vi "Generate Non-Linear X-component.vi"(7 "Current Calibration Type":T1, 9 "Reso Phase correction factor":dbl, 10 "Start Delay (Ticks)":dbl, 11 "X Pixel Dimension":i32) -> (3 "Non-Linear X pixel Distribution (Linear for Galvo)":dbl[](array[numeric]))   [LabVIEW 2012]
uses:
  Custom Controls and Typedefs/CalibrationType.ctl
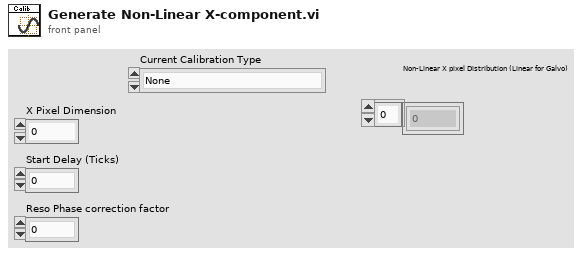
[diagram p1: front panel]
types:
  T1 = typedef "CalibrationType.ctl" = enum16{"None", "ImagingGalvoCalibration", "ImagingResoCalibration"}
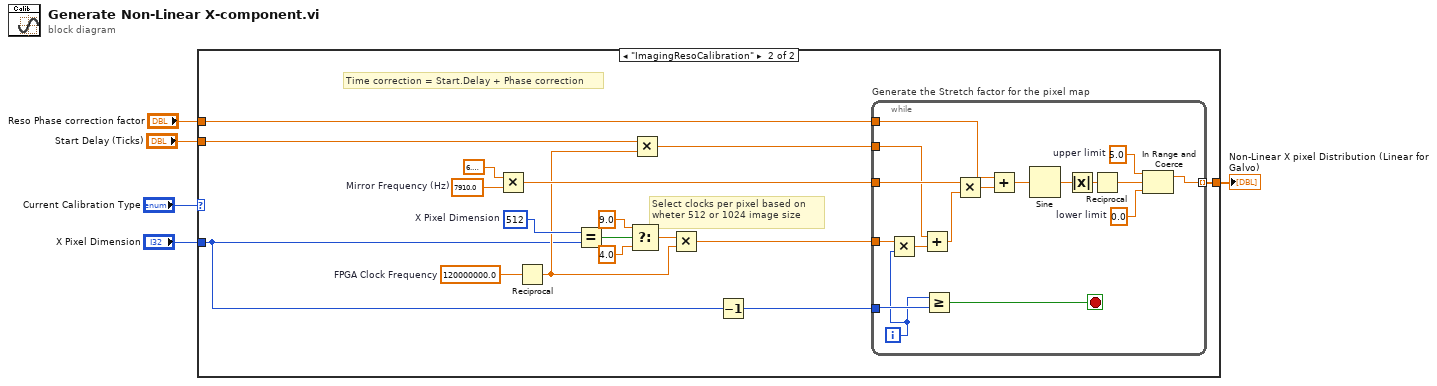
[diagram p0: block diagram]
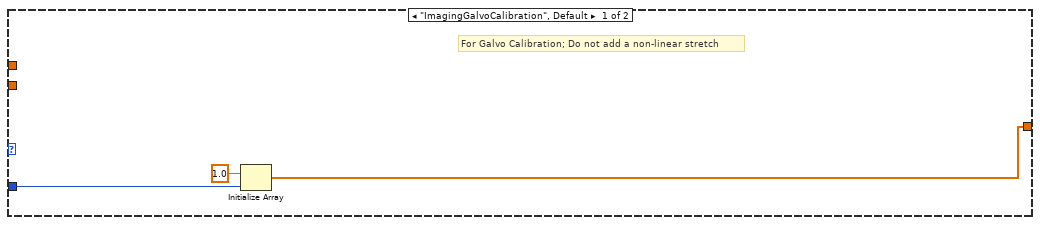
[diagram p2: hidden frame]
diagram:
  n1 = case shown="\"ImagingResoCalibration\"" "Current Calibration Type" {
    tunnel: [w7 w12] -> w3
    tunnel: "X Pixel Dimension" -> [w6 w11]
    tunnel: "Reso Phase correction factor" -> [_ w10]
    tunnel: "Start Delay (Ticks)" -> [_ w9]
    frame "ImagingGalvoCalibration", Default {
      # "For Galvo Calibration; Do not add a non-linear stretch"
      n2 = Initialize Array(1.0 ("upper limit"), w6) -> (w7:dbl[])
    }
    frame "ImagingResoCalibration" {
      w16 = 512  # X Pixel Dimension
      w22 = 120000000.0  # FPGA Clock Frequency
      w23 = 7910.0  # Mirror Frequency (Hz)
      # "Time correction = Start.Delay + Phase correction"
      # "Select clocks per pixel based on wheter 512 or 1024 image size"
      n3 = Multiply(x=6.283185307179586, y=w23) -> (x*y=w24:dbl)
      n4 = Reciprocal(x=w22) -> (1/x=w14:dbl)
      n5 = Equal?(x=w16, y=w11) -> (x = y?=w20:bool)
      n6 = Select(t=9.0 ("clocks per pixel"), s=w20, f=4.0) -> (s? t:f=w15:dbl)
      n7 = Multiply(x=w9, y=w14) -> (x*y=w13:dbl)
      n8 = Multiply(x=w15, y=w14) -> (x*y=w21:dbl)
      n9 = Decrement(x=w11) -> (x-1=w17:i32)
      n10 = while "Generate the Stretch factor for the pixel map" {
        tunnel: w21 -> [w42]
        tunnel: w24 -> [w41]
        tunnel: [w26] -> w12 mode=indexing
        tunnel: w17 -> [w38]
        tunnel: w13 -> [w34]
        tunnel: w10 -> [w31]
        i -> [w36]
        stop <- w37 stop-if-true
        w27 = 5.0  # upper limit
        w28 = 0.0  # lower limit
        n11 = Multiply(x=w42, y=w36) -> (x*y=w35:dbl)
        n12 = Add(x=w34, y=w35) -> (x+y=w33:dbl)
        n13 = Greater Or Equal?(x=w36, y=w38) -> (x >= y?=w37:bool)
        n14 = Multiply(x=w41, y=w33) -> (x*y=w32:dbl)
        n15 = Add(x=w31, y=w32) -> (x+y=w30:dbl)
        n16 = Sine(x=w30) -> (sin(x)=w40:dbl)
        n17 = Absolute Value(x=w40) -> (abs(x)=w39:dbl)
        n18 = Reciprocal(x=w39) -> (1/x=w29:dbl)
        n19 = In Range and Coerce(upper limit=w27, x=w29, lower limit=w28) -> (coerced(x)=w26:dbl)  [unwired: 1 out]
      }
    }
  }
  "Non-Linear X pixel Distribution (Linear for Galvo)" <- w3
